vi "FTW-Endpoint-Multipart-Receive.vi"(0 "FTW Endpoint":refnum<class "FTW-Endpoint-TCP.lvclass">, 5 "Timeout":i32 format="%dmsec", 11 "error in":errorcluster) -> (4 "FTW Endpoint out":refnum<class "FTW-Endpoint-TCP.lvclass">, 6 "Message Received":string[](array[string]), 8 "Timed out?":bool, 15 "error out":errorcluster)   [LabVIEW 2013, in "FTW-Endpoint-TCP.lvclass"]
uses:
  FTW-Endpoint-TCP.lvclass
  FTW-Endpoint-TCP.lvclass/FTW-Endpoint-TCP.ctl
  Core/src/Error/FTW-ERR-Clear.vi
panel:
  # "Inputs"
  # "Outputs"
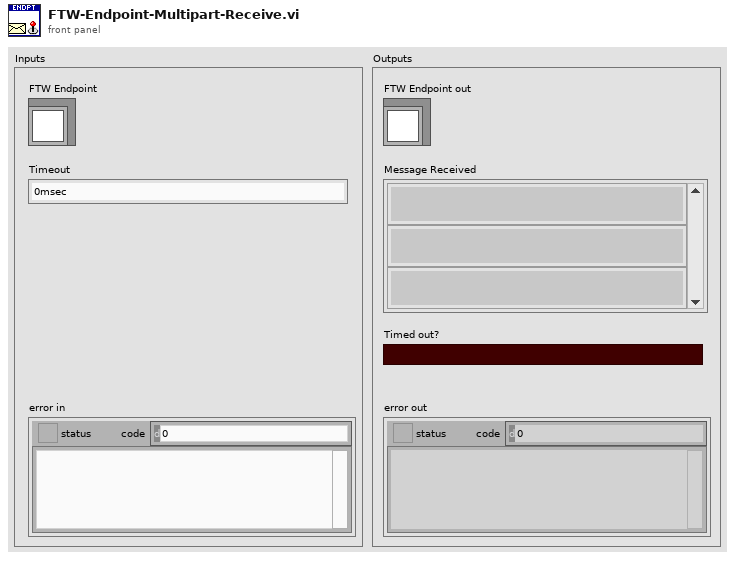
[diagram p1: front panel]
types:
  T1 = enum16{"Standard", "Buffered", "CRLF", "Immediate"}
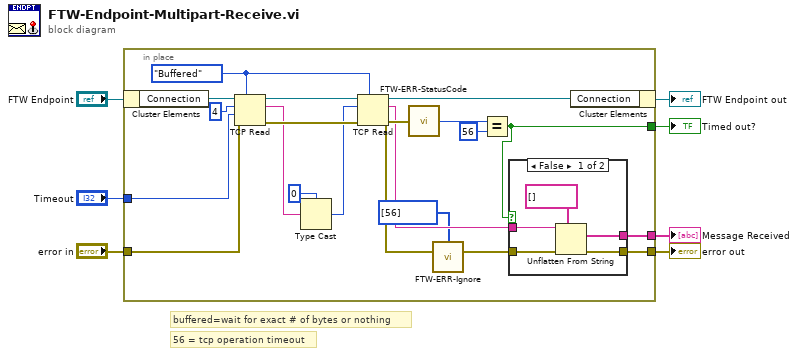
[diagram p0: block diagram]
diagram:
  # "56 = tcp operation timeout"
  # "buffered=wait for exact # of bytes or nothing"
  n1 = in-place {
    in-place-border: [w16] -> w7
    in-place-border: "error in" -> [w19]
    in-place-border: "Timeout" -> [w18]
    in-place-border: [w13] -> w2
    in-place-border: [w10] -> w1
    w21 = T1."Buffered" ("mode (standard)")
    n2 = in-place-cluster #1("FTW Endpoint") -> ("Connection"=w20:refnum<k5>)
    n3 = TCP Read(connection ID=w20, bytes to read=4, error in (no error)=w19, 7:w21, 9:w18) -> (connection ID out=w25:refnum<k5>, data out=w24:string, error out=w26:errorcluster)
    n4 = Type Cast(type=0, x=w24) -> (*(type *) &x=w22:i32)
    n5 = TCP Read(connection ID=w25, bytes to read=w22, error in (no error)=w26, 7:w21) -> (connection ID out=w17:refnum<k5>, data out=w12:string, error out=w15:errorcluster)  [unwired: 1 in]
    n6 = call "FTW-ERR-StatusCode.vi"("error to check"=w15) -> ("Code"=w14:i32)
    n7 = call "FTW-ERR-Ignore.vi"("Codes to filter"=i32[] [56], "error to filter"=w15) -> ("filtered error"=w9:errorcluster)  [unwired: 13 in]
    n8 = Equal?(x=w14, y=56 ("x")) -> (x = y?=w10:bool)
    n9 = case shown="False" w10 {
      tunnel: [w32 w33] -> w16
      tunnel: w9 -> [w30 w33]
      tunnel: [w29 _] -> w13
      tunnel: w12 -> [w28 _]
      frame False {
        n10 = Unflatten From String(type=string[] [], binary string=w28, error in (no error)=w30) -> (value=w29:string[], error out=w32:errorcluster)  [unwired: 2 in, 1 out]
      }
      frame True {
      }
    }
    n11 = in-place-cluster #1("Connection"=w17) -> (→"FTW Endpoint out":refnum<class "FTW-Endpoint-TCP.lvclass">)
  }
  "error out" <- w7
  "Message Received" <- w2
  "Timed out?" <- w1
